vi "move_1ax_thor_z825b_2.vi"(11 "fAbsPosCh2":sgl) -> ()   [LabVIEW 2013]
panel:
  out "pfPosition":sgl
  out "error out":errorcluster
  in  "serial":i32
  in  "MG17Motor":refnum<k7>(container)
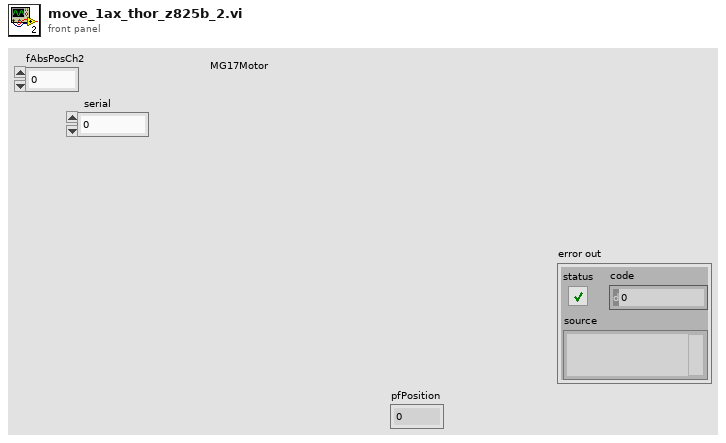
[diagram p1: front panel]
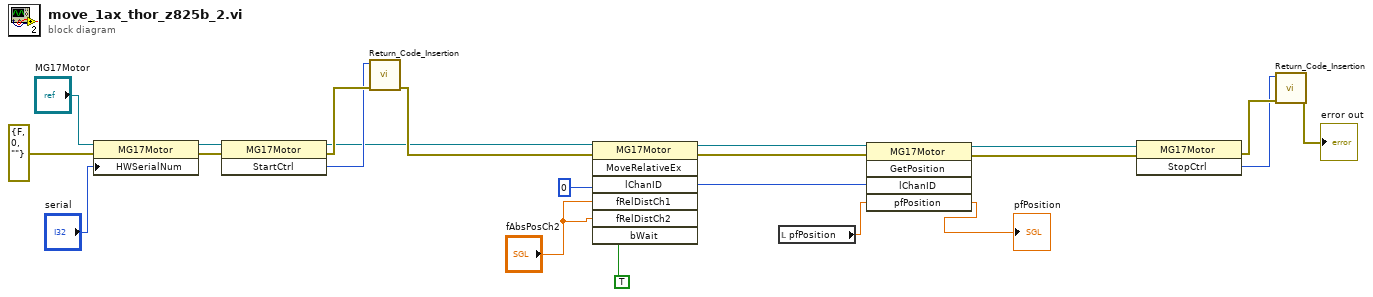
[diagram p0: block diagram]
diagram:
  n1 = property class="MG17Motor"(reference="MG17Motor", error in=errorcluster {"status"=FALSE, "code"=0, "source"=""} ("error in (no error)"), "HWSerialNum"="serial") -> (reference out=w20:refnum<k7>, error out=w18:errorcluster)
  n2 = invoke class="MG17Motor" method="StartCtrl"(reference=w20, error in=w18) -> (reference out=w6:refnum<k7>, error out=w17:errorcluster, "StartCtrl"=w16:i32)  [unwired: 1 in]
  n3 = call "Return_Code_Insertion.vi"("error in (no error)"=w17, "Return Code"=w16) -> ("error out"=w7:errorcluster)  [unwired: 9 in]
  n4 = invoke class="MG17Motor" method="MoveRelativeEx"(reference=w6, error in=w7, "lChanID"=0, "fRelDistCh1"="fAbsPosCh2", "fRelDistCh2"="fAbsPosCh2", "bWait"=TRUE) -> (reference out=w4:refnum<k7>, error out=w5:errorcluster, "lChanID"=w1:i32)  [unwired: 1 in, 4 out]
  n5 = local read "pfPosition"() -> (w11:sgl)
  n6 = invoke class="MG17Motor" method="GetPosition"(reference=w4, error in=w5, "lChanID"=w1, "pfPosition"=w11) -> (reference out=w2:refnum<k7>, error out=w3:errorcluster, "pfPosition"=→"pfPosition":sgl)  [unwired: 1 in, 2 out]
  n7 = invoke class="MG17Motor" method="StopCtrl"(reference=w2, error in=w3) -> (error out=w15:errorcluster, "StopCtrl"=w14:i32)  [unwired: 1 in, 1 out]
  n8 = call "Return_Code_Insertion.vi"("error in (no error)"=w15, "Return Code"=w14) -> ("error out"=→"error out":errorcluster)  [unwired: 9 in]
